vi "Close.vi"(8 "error in":errorcluster, 11 "Config from XML in":refnum<class "Config from XML.lvclass">) -> (0 "error out":errorcluster, 3 "Config from XML out":refnum<class "Config from XML.lvclass">)   [LabVIEW 2019, in "Configuration.lvlib" / "Config from XML.lvclass"]
uses:
  Config from XML.lvclass
  Config from XML.lvclass/Config from XML.ctl
  <vilib>/xml/NI_XML.lvlib
  <vilib>/xml/Close Reference(Node).vi
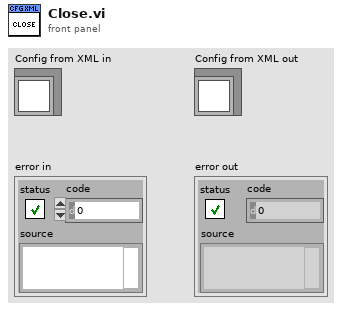
[diagram p1: front panel]
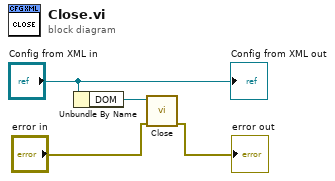
[diagram p0: block diagram]
diagram:
  n1 = Unbundle By Name("Config from XML in") -> ("DOM"=w3:refnum<k20>)
  n2 = call-poly <vilib>:"Close.vi"("error in (no error)"="error in", "node"=w3) -> ("error out"=→"error out":errorcluster)  [unwired: 7 out]
  "Config from XML out" <- "Config from XML in"
